vi "Compute (Array).vi"(8 "error in (no error)":errorcluster, 10 "Data Points in":T1, 11 "Aux Data Source in":refnum<class "Aux Data Source.lvclass">) -> (0 "error out":errorcluster, 2 "Data Points out":T1, 3 "Aux Data Source out":refnum<class "Aux Data Source.lvclass">)   [LabVIEW 2017, in "Aux Data Source.lvclass"]
doc: "Process and return an array of data points at the end of a scan. (For example, to normalize the output or find min/max, one must know all data points a priori.)"
uses:
  Aux Data Source.lvclass
  Instruments/Utility Classes/Readable/Data Points.ctl
  Instruments/Utility Classes/Readable/Data Point.ctl
  Instruments/Utility Classes/Readable/Time.ctl
  Instruments/Utility Classes/Readable/X.ctl
  Instruments/Utility Classes/Readable/Readable.lvclass
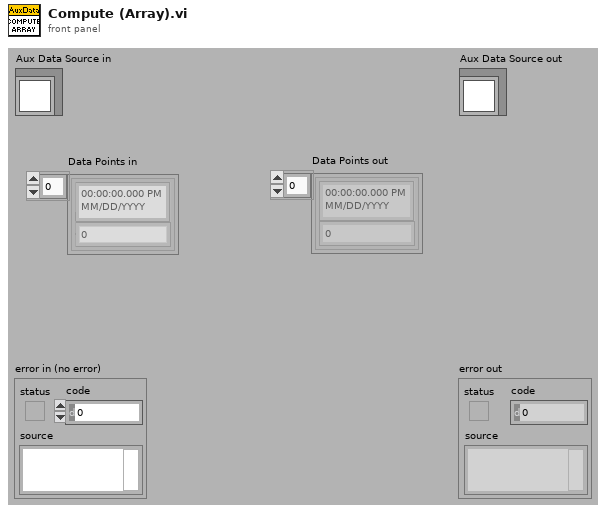
[diagram p1: front panel]
types:
  T1 = typedef "Readable.lvclass/Data Points.ctl" = T2[]
  T2 = typedef "Readable.lvclass/Data Point.ctl" = cluster{"t":T3, "x":T4}
  T3 = typedef "Readable.lvclass/Time.ctl" = timestamp
  T4 = typedef "Readable.lvclass/X.ctl" = dbl
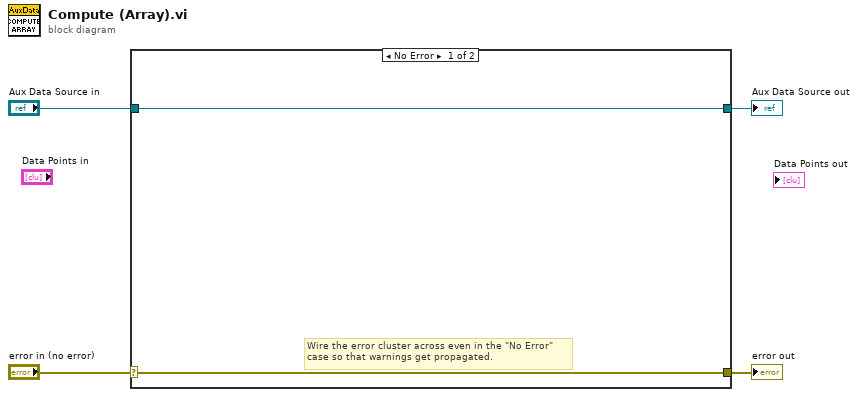
[diagram p0: block diagram]
diagram:
  n1 = case shown="No Error" "error in (no error)" {
    selector: "error in (no error)" -> [w5 w8]
    tunnel: [w5 w8] -> w3
    tunnel: [w6 w7] -> w1
    tunnel: "Aux Data Source in" -> [w6 w7]
    frame No Error {
      # "Wire the error cluster across even in the \"No Error\"\ncase so that warnings get propagated."
    }
    frame Error {
    }
  }
  "error out" <- w3
  "Aux Data Source out" <- w1
